vi "Priority.vi"(8 "error in (no error)":errorcluster, 11 "Caching Response in":refnum<class "Caching Response.lvclass">) -> (0 "error out":errorcluster, 2 "Priority":u16, 3 "Caching Response out":refnum<class "Caching Response.lvclass">)   [LabVIEW 2020, in "HTTP Server.lvlib" / "Caching Response.lvclass"]
uses:
  Caching Response.lvclass
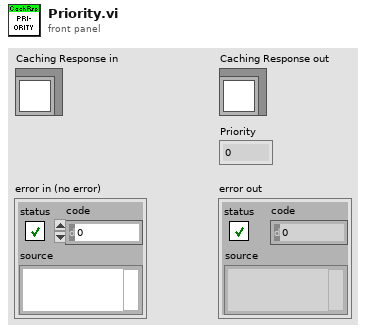
[diagram p1: front panel]
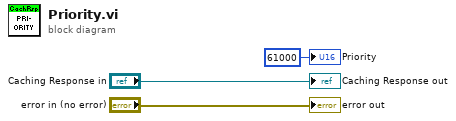
[diagram p0: block diagram]
diagram:
  "error out" <- "error in (no error)"
  "Caching Response out" <- "Caching Response in"
  "Priority" <- u16 61000 ("Priority")
